vi "final16_working_not_in_order.vi"() -> ()   [LabVIEW 2019]
uses:
  <vilib>/Instr/_visa.llb/VISA Configure Serial Port (Instr).vi
  <vilib>/Utility/file.llb/Write Delimited Spreadsheet (DBL).vi
  <vilib>/Analysis/NI_AALBase.lvlib
  <vilib>/Analysis/NI_AALPro.lvlib
panel:
  out "intercept_gain2":dbl
  out "slope_gain2":dbl
  out "intercept_gain1":dbl
  out "slope_gain1":dbl
  out "intercept_gain0":dbl
  out "slope_gain0":dbl
  out "Conversion [g]":dbl
  out "Debug array":string[](array[string])
  in  "Stop":bool
  in  "Cycles":dbl min=1.0 step=1.0
  in  "Start operation":bool
  out "String passed to Arduino":string
  in  "Function":u16(ring) items=["Read data ", "Compare different gains", "Execute calibration"]
  out "Received data":string
  in  "Gain":u16(ring) items=["32", "64", "128"]
  out "mean":dbl format="%0.2f"
  out "variance":dbl format="%0.2f"
  out "standard deviation":dbl format="%0.2f"
  in  "Save data path":path
  in  "Arduino COM port":refnum<visa-resource-name>="COM6"
  # "Select all options, then press \"Start operation\" button"
  # "Nerd zone"
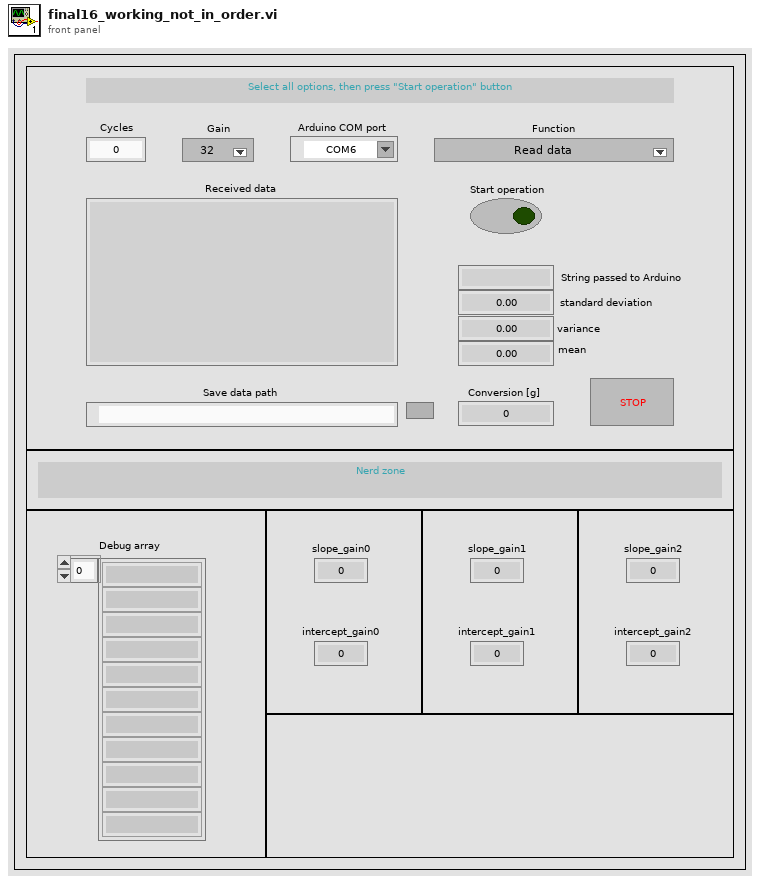
[diagram p1: front panel]
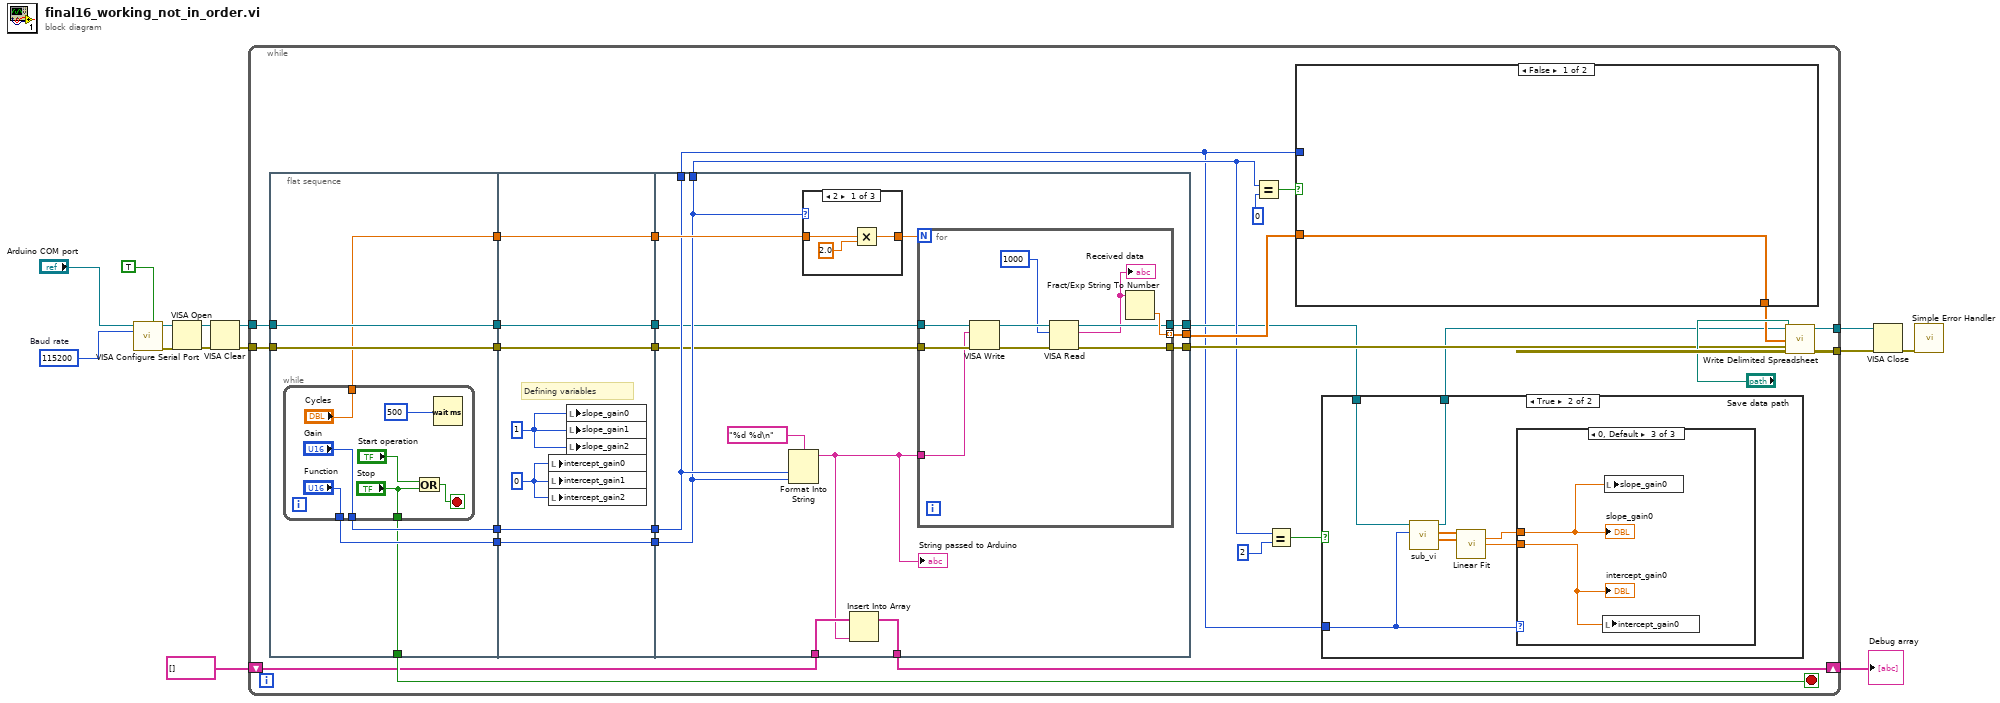
[diagram p0: block diagram]
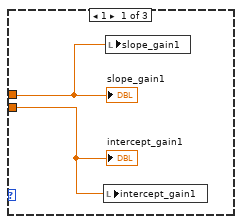
[diagram p3: hidden frame]
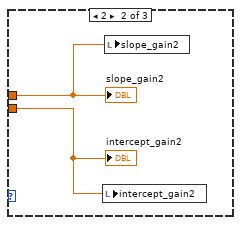
[diagram p4: hidden frame]
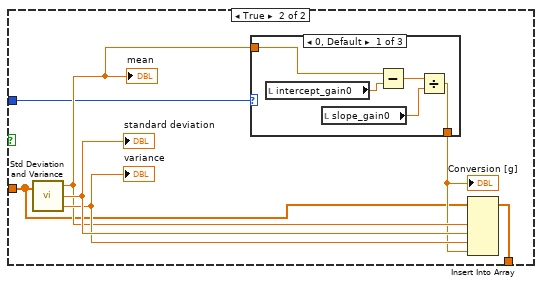
[diagram p5: hidden frame]
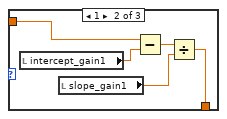
[diagram p6: hidden frame]
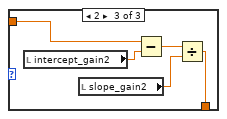
[diagram p7: hidden frame]
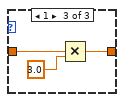
[diagram p9: hidden frame]
diagram:
  w13 = u32 115200  # Baud rate
  n1 = call-poly "VISA Configure Serial Port"("VISA resource name"="Arduino COM port", "Enable Termination\nChar (T)"=TRUE ("Enable Termination\nChar (T)"), "baud rate (9600)"=w13) -> ("VISA resource name out"=w11:refnum<visa-resource-name>, "error out"=w12:errorcluster)  [unwired: 11 in]
  n2 = VISA Open(error in (no error)=w12, VISA resource name=w11) -> (VISA resource name=w8:refnum<visa-resource-name>, error out=w9:errorcluster)  [unwired: 3 in]
  n3 = VISA Clear(VISA resource name=w8, error in (no error)=w9) -> (VISA resource name out=w6:refnum<visa-resource-name>, error out=w7:errorcluster)
  n4 = while {
    tunnel: w7 -> [w42]
    tunnel: w6 -> [w41]
    shift-right: [w40] -> w4
    shift-left: string[] [] -> [w36]
    tunnel: [w37] -> w3
    tunnel: [w26] -> w1
    stop <- w39 stop-if-true
    n5 = flat-sequence {
      tunnel: [w85] -> w22
      tunnel: [w84] -> w24
      tunnel: [w83] -> w20
      tunnel: [w82] -> w18
      tunnel: w42 -> [w84]
      tunnel: w41 -> [w85]
      tunnel: [w81] -> w16
      tunnel: [w80] -> w39
      tunnel: w24 -> [w99]
      tunnel: [w99] -> w23
      tunnel: w22 -> [w98]
      tunnel: [w98] -> w21
      tunnel: w20 -> [w97]
      tunnel: [w97] -> w19
      tunnel: w18 -> [w96]
      tunnel: [w96] -> w17
      tunnel: w16 -> [w95]
      tunnel: [w95] -> w15
      tunnel: [w112] -> w27
      tunnel: [w111] -> w29
      tunnel: [w110] -> w34
      tunnel: w23 -> [w100]
      tunnel: w21 -> [w101]
      tunnel: w19 -> [w102]
      tunnel: w17 -> [w103]
      tunnel: w15 -> [w107]
      tunnel: [w104] -> w40
      tunnel: w36 -> [w106]
      tunnel: [w103] -> w25
      tunnel: [w102] -> w28
      frame #0 {
        n6 = while {
          tunnel: ["Function"] -> w83
          tunnel: ["Gain"] -> w82
          tunnel: ["Cycles"] -> w81
          tunnel: ["Stop"] -> w80
          stop <- w87 stop-if-true
          n7 = Or(x="Start operation", y="Stop") -> (x .or. y?=w87:bool)
          n8 = Wait (ms)(milliseconds to wait=u32 500) -> ()  [unwired: 1 out]
        }
      }
      frame #1 {
        w93 = 0
        w94 = 1
        # "Defining variables"
        n9 = local write "intercept_gain0"(w93) -> ()
        n10 = local write "intercept_gain1"(w93) -> ()
        n11 = local write "intercept_gain2"(w93) -> ()
        n12 = local write "slope_gain0"(w94) -> ()
        n13 = local write "slope_gain1"(w94) -> ()
        n14 = local write "slope_gain2"(w94) -> ()
      }
      frame #2 {
        n15 = Format Into String(format string="%d %d\n", w103, w102) -> (resulting string=w105:string)  [unwired: 2 in, 1 out]
        "String passed to Arduino" <- w105
        n16 = case shown="2" w102 {
          tunnel: w107 -> [w115 w116 w117]
          tunnel: [w113 w116 w118] -> w108
          frame 2 {
            n17 = Multiply(x=w115, y=2.0) -> (x*y=w113:dbl)
          }
          frame 0, Default {
          }
          frame 1 {
            n18 = Multiply(x=w117, y=3.0) -> (x*y=w118:dbl)
          }
        }
        n19 = Insert Into Array(array=w106, new element=w105) -> (w104:string[])  [unwired: 1 in]
        n20 = for {
          N: w108 -> [_]
          tunnel: [w124] -> w110 mode=indexing
          tunnel: w105 -> [w120]
          tunnel: w101 -> [w126]
          tunnel: [w123] -> w112
          tunnel: w100 -> [w127]
          tunnel: [w125] -> w111
          n21 = VISA Write(VISA resource name=w126, write buffer=w120, error in (no error)=w127) -> (VISA resource name out=w129:refnum<visa-resource-name>, error out=w128:errorcluster)  [unwired: 1 out]
          n22 = VISA Read(VISA resource name=w129, byte count=u32 1000, error in (no error)=w128) -> (VISA resource name out=w123:refnum<visa-resource-name>, read buffer=w122:string, error out=w125:errorcluster)  [unwired: 1 out]
          "Received data" <- w122
          n23 = Fract/Exp String To Number(string=w122) -> (number=w124:dbl)  [unwired: 3 in, 1 out]
        }
      }
    }
    n24 = Equal?(x=w28, y=u16 0) -> (x = y?=w33:bool)
    n25 = Equal?(x=w28, y=u16 2) -> (x = y?=w30:bool)
    n26 = case shown="False" w33 {
      tunnel: [w57 w62] -> w35
      tunnel: w34 -> [w57 w59]
      tunnel: w25 -> [_ w58]
      frame False {
      }
      frame True {
        n27 = call <vilib>:"Std Deviation and Variance.vi"("X"=w59) -> ("mean"=w61:dbl, "standard deviation"=w64:dbl, "variance"=w63:dbl)  [unwired: 1 in]
        "standard deviation" <- w64
        "variance" <- w63
        "mean" <- w61
        n28 = case shown="0, Default" w58 {
          tunnel: w61 -> [w69 w72 w77]
          tunnel: [w67 w73 w78] -> w60
          frame 0, Default {
            n29 = local read "intercept_gain0"() -> (w65:dbl)
            n30 = local read "slope_gain0"() -> (w66:dbl)
            n31 = Subtract(x=w69, y=w65) -> (x-y=w68:dbl)
            n32 = Divide(x=w68, y=w66) -> (x/y=w67:dbl)
          }
          frame 1 {
            n33 = local read "intercept_gain1"() -> (w71:dbl)
            n34 = local read "slope_gain1"() -> (w70:dbl)
            n35 = Subtract(x=w72, y=w71) -> (x-y=w74:dbl)
            n36 = Divide(x=w74, y=w70) -> (x/y=w73:dbl)
          }
          frame 2 {
            n37 = local read "intercept_gain2"() -> (w76:dbl)
            n38 = local read "slope_gain2"() -> (w75:dbl)
            n39 = Subtract(x=w77, y=w76) -> (x-y=w79:dbl)
            n40 = Divide(x=w79, y=w75) -> (x/y=w78:dbl)
          }
        }
        "Conversion [g]" <- w60
        n41 = Insert Into Array(array=w59, new element #1=w61, new element #2=w64, new element #3=w63, new element #4=w60) -> (w62:dbl[])  [unwired: 1 in]
      }
    }
    n42 = case shown="True" w30 {
      tunnel: w25 -> [_ w46]
      tunnel: w27 -> [w43 w48]
      tunnel: [w43 w47] -> w26
      frame False {
      }
      frame True {
        n43 = call "sub_vi.vi"("Gain"=w46, "VISA resource name"=w48) -> ("Weights"=w49:dbl[], "Measures"=w50:dbl[], "VISA resource name out"=w47:refnum<visa-resource-name>)  [unwired: 6 in, 1 out]
        n44 = call <vilib>:"Linear Fit.vi"("Y"=w50, "X"=w49) -> ("slope"=w45:dbl, "intercept"=w44:dbl)  [unwired: 9 in, 3 out]
        n45 = case shown="0, Default" w46 {
          tunnel: w45 -> [w52 w54 w56]
          tunnel: w44 -> [w51 w53 w55]
          frame 1 {
            n46 = local write "intercept_gain1"(w51) -> ()
            n47 = local write "slope_gain1"(w52) -> ()
            "slope_gain1" <- w52
            "intercept_gain1" <- w51
          }
          frame 2 {
            n48 = local write "intercept_gain2"(w53) -> ()
            n49 = local write "slope_gain2"(w54) -> ()
            "slope_gain2" <- w54
            "intercept_gain2" <- w53
          }
          frame 0, Default {
            n50 = local write "intercept_gain0"(w55) -> ()
            n51 = local write "slope_gain0"(w56) -> ()
            "slope_gain0" <- w56
            "intercept_gain0" <- w55
          }
        }
      }
    }
    n52 = call-poly <vilib>:"Write Delimited Spreadsheet.vi"("file path (dialog if empty)"="Save data path", "1D data"=w35, "error in (no error)"=w29) -> ("error out"=w37:errorcluster)  [unwired: 11 in, 1 out]
  }
  "Debug array" <- w4
  n53 = VISA Close(VISA resource name=w1, error in (no error)=w3) -> (error out=w2:errorcluster)
  n54 = call <vilib>:"Simple Error Handler.vi"("error in (no error)"=w2) -> ()  [unwired: 4 in, 5 out]
